vi "hcam_parse_packet.vi"(7 "packet data":u8[](array[numeric])) -> (8 "sensor data out":T1)   [LabVIEW 2020]
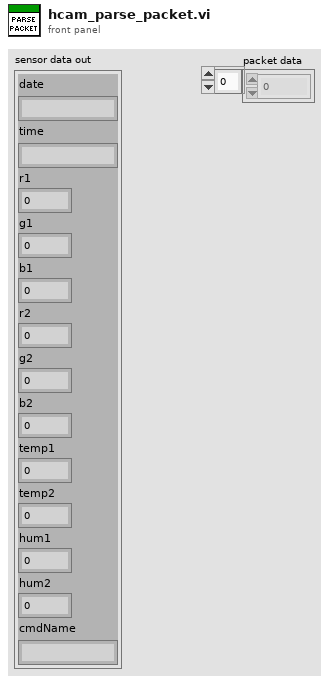
[diagram p1: front panel]
types:
  T1 = cluster{"date":string, "time":string, "r1":u8, "g1":u8, "b1":u8, "r2":u8, "g2":u8, "b2":u8, "temp1":sgl, "temp2":sgl, "hum1":sgl, "hum2":sgl, "cmdName":string}
  T2 = cluster{"index":u8, "length":u8, "type":string}[]
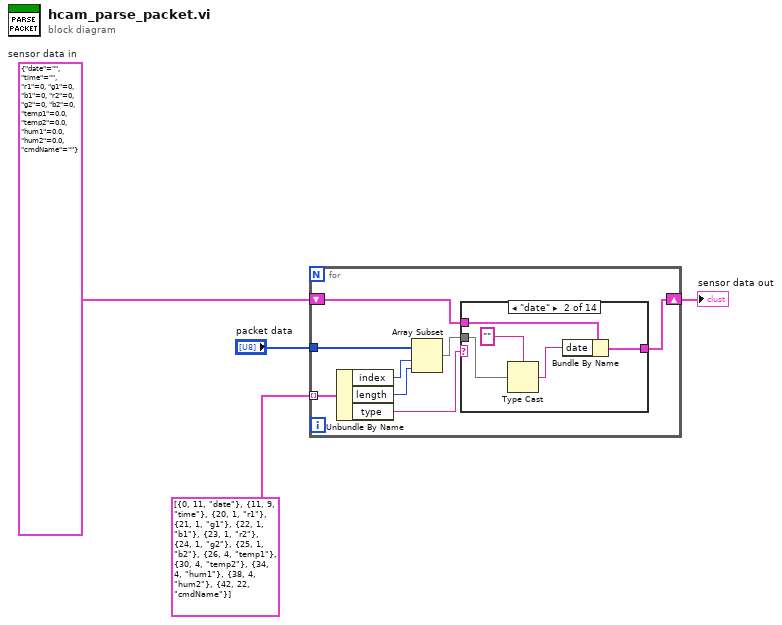
[diagram p0: block diagram]
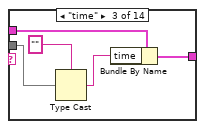
[diagram p3: hidden frame]
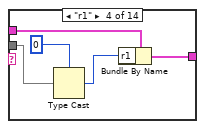
[diagram p4: hidden frame]
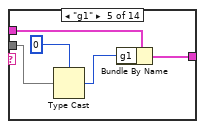
[diagram p5: hidden frame]
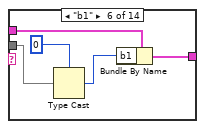
[diagram p6: hidden frame]
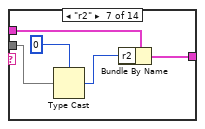
[diagram p7: hidden frame]
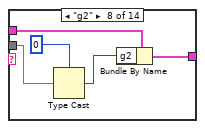
[diagram p8: hidden frame]
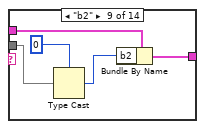
[diagram p9: hidden frame]
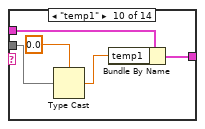
[diagram p10: hidden frame]
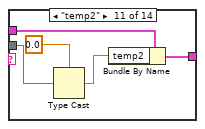
[diagram p11: hidden frame]
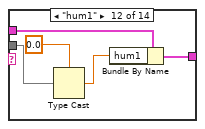
[diagram p12: hidden frame]
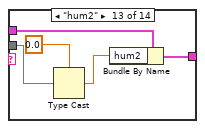
[diagram p13: hidden frame]
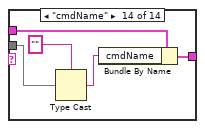
[diagram p14: hidden frame]
diagram:
  w2 = T1 {"date"="", "time"="", "r1"=0, "g1"=0, "b1"=0, "r2"=0, "g2"=0, "b2"=0, "temp1"=0.0, "temp2"=0.0, "hum1"=0.0, "hum2"=0.0, "cmdName"=""}  # sensor data in
  n1 = for {
    tunnel: "packet data" -> [w12]
    tunnel: T2 [{"index"=0, "length"=11, "type"="date"}, {"index"=11, "length"=9, "type"="time"}, {"index"=20, "length"=1, "type"="r1"}, {"index"=21, "length"=1, "type"="g1"}, {"index"=22, "length"=1, "type"="b1"}, {"index"=23, "length"=1, "type"="r2"}, {"index"=24, "length"=1, "type"="g2"}, {"index"=25, "length"=1, "type"="b2"}, {"index"=26, "length"=4, "type"="temp1"}, {"index"=30, "length"=4, "type"="temp2"}, {"index"=34, "length"=4, "type"="hum1"}, {"index"=38, "length"=4, "type"="hum2"}, {"index"=42, "length"=22, "type"="cmdName"}] ("packet decimation") -> [w11] mode=indexing
    shift-right: [w5] -> w1
    shift-left: w2 -> [w6]
    n2 = Unbundle By Name(w11) -> ("index"=w10:u8, "length"=w9:u8, "type"=w8:string)
    n3 = Array Subset(array=w12, index=w10, length=w9) -> (w7:u8[])
    n4 = case shown="\"date\"" w8 {
      tunnel: w7 -> [_ w17 w22 w27 w32 w37 w42 w47 w52 w57 w62 w67 w72 w77]
      tunnel: w6 -> [w13 w16 w21 w26 w31 w36 w41 w46 w51 w56 w61 w66 w71 w76]
      tunnel: [w13 w14 w19 w24 w29 w34 w39 w44 w49 w54 w59 w64 w69 w74] -> w5
      frame Default {
      }
      frame "date" {
        n5 = Type Cast(type="", x=w17) -> (*(type *) &x=w15:string)
        n6 = Bundle By Name(cluster=w16, "date"=w15) -> (w14:T1)
      }
      frame "time" {
        n7 = Type Cast(type="", x=w22) -> (*(type *) &x=w20:string)
        n8 = Bundle By Name(cluster=w21, "time"=w20) -> (w19:T1)
      }
      frame "r1" {
        n9 = Type Cast(type=u8 0, x=w27) -> (*(type *) &x=w25:u8)
        n10 = Bundle By Name(cluster=w26, "r1"=w25) -> (w24:T1)
      }
      frame "g1" {
        n11 = Type Cast(type=u8 0, x=w32) -> (*(type *) &x=w30:u8)
        n12 = Bundle By Name(cluster=w31, "g1"=w30) -> (w29:T1)
      }
      frame "b1" {
        n13 = Type Cast(type=u8 0, x=w37) -> (*(type *) &x=w35:u8)
        n14 = Bundle By Name(cluster=w36, "b1"=w35) -> (w34:T1)
      }
      frame "r2" {
        n15 = Type Cast(type=u8 0, x=w42) -> (*(type *) &x=w40:u8)
        n16 = Bundle By Name(cluster=w41, "r2"=w40) -> (w39:T1)
      }
      frame "g2" {
        n17 = Type Cast(type=u8 0, x=w47) -> (*(type *) &x=w45:u8)
        n18 = Bundle By Name(cluster=w46, "g2"=w45) -> (w44:T1)
      }
      frame "b2" {
        n19 = Type Cast(type=u8 0, x=w52) -> (*(type *) &x=w50:u8)
        n20 = Bundle By Name(cluster=w51, "b2"=w50) -> (w49:T1)
      }
      frame "temp1" {
        n21 = Type Cast(type=sgl 0.0, x=w57) -> (*(type *) &x=w55:sgl)
        n22 = Bundle By Name(cluster=w56, "temp1"=w55) -> (w54:T1)
      }
      frame "temp2" {
        n23 = Type Cast(type=sgl 0.0, x=w62) -> (*(type *) &x=w60:sgl)
        n24 = Bundle By Name(cluster=w61, "temp2"=w60) -> (w59:T1)
      }
      frame "hum1" {
        n25 = Type Cast(type=sgl 0.0, x=w67) -> (*(type *) &x=w65:sgl)
        n26 = Bundle By Name(cluster=w66, "hum1"=w65) -> (w64:T1)
      }
      frame "hum2" {
        n27 = Type Cast(type=sgl 0.0, x=w72) -> (*(type *) &x=w70:sgl)
        n28 = Bundle By Name(cluster=w71, "hum2"=w70) -> (w69:T1)
      }
      frame "cmdName" {
        n29 = Type Cast(type="", x=w77) -> (*(type *) &x=w75:string)
        n30 = Bundle By Name(cluster=w76, "cmdName"=w75) -> (w74:T1)
      }
    }
  }
  "sensor data out" <- w1
